vi "Thumper Control.vi"(11 "Thump":bool) -> ()   [LabVIEW 2016]
uses:
  <vilib>/Rock Robotics/Network Tables/NT Read Number.vi
  <vilib>/Rock Robotics/WPI/Solenoid/WPI_SolenoidSetEnum.vi
  <vilib>/Rock Robotics/WPI/Solenoid/Deprecated/WPI_SolenoidGetBool.vi
panel:
  in  "Thumper Status":bool
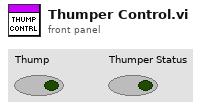
[diagram p1: front panel]
types:
  T1 = typedef "WPI_SolenoidDevRef.ctl" = cluster{"DevStatus":errorcluster, "Pneumatics Control Module":u8, "Forward Solenoid Channel":T2, "Reverse Solenoid Channel":T2}
  T2 = typedef "WPI_SolenoidChannel.ctl" = enum8{"Solenoid 0", "Solenoid 1", "Solenoid 2", "Solenoid 3", "Solenoid 4", "Solenoid 5", "Solenoid 6", "Solenoid 7", "Invalid"}
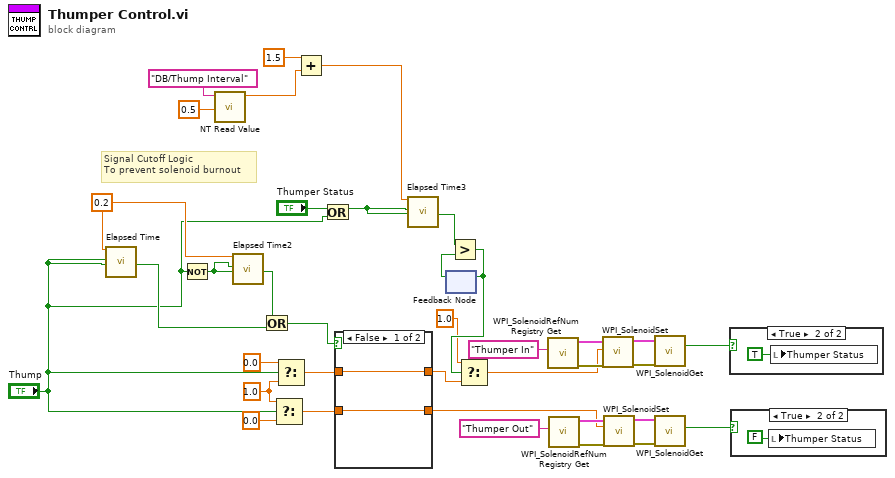
[diagram p0: block diagram]
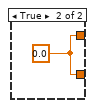
[diagram p4: hidden frame]
diagram:
  w31 = 0.2 ("Time Target (s)")
  w26 = 1.0 ("f")
  # "Signal Cutoff Logic\nTo prevent solenoid burnout"
  n1 = call "Elapsed Time"("Time Target (s)"=w31, "Reset"="Thump", "Auto Reset"="Thump") -> ("Time has Elapsed"=w28:bool)  [unwired: 9 in, 7 out]
  n2 = Not(x="Thump") -> (.not. x?=w30:bool)
  n3 = call-poly <vilib>:"NT Read Value.vi"("Default Value"=0.5, "Name"="DB/Thump Interval") -> ("Numeric"=w5:dbl)  [unwired: 8 in, 1 out]
  n4 = call "Elapsed Time2"("Time Target (s)"=w31, "Reset"=w30, "Auto Reset"=w30) -> ("Time has Elapsed"=w29:bool)  [unwired: 9 in, 7 out]
  n5 = Or(x=w29, y=w28) -> (x .or. y?=w27:bool)
  n6 = Select(t=w26, s="Thump", f=0.0) -> (s? t:f=w24:dbl)
  n7 = Select(t=0.0, s="Thump", f=w26) -> (s? t:f=w23:dbl)
  n8 = Add(x=1.5 ("Time Target (s)"), y=w5) -> (x+y=w4:dbl)
  n9 = Or(x="Thumper Status", y="Thump") -> (x .or. y?=w2:bool)
  n10 = case shown="False" w27 {
    tunnel: [w39 w40] -> w25
    tunnel: w24 -> [w39 _]
    tunnel: [w38 w40] -> w13
    tunnel: w23 -> [w38 _]
    frame False {
    }
    frame True {
      w40 = 0.0 ("f")
    }
  }
  n11 = call "Elapsed Time3"("Time Target (s)"=w4, "Reset"=w2, "Auto Reset"=w2) -> ("Time has Elapsed"=w12:bool)  [unwired: 9 in, 7 out]
  n12 = feedback #1() -> (w11:bool)  [unwired: 1 in]
  n13 = Greater?(x=w12, y=w11) -> (0:w10:bool)
  n14 = feedback-in #1(w10) -> ()
  n15 = Select(t=1.0, s=w10, f=w13) -> (s? t:f=w14:dbl)
  n16 = call <vilib>:"WPI_SolenoidRefNum Registry Get.vi"("refnum name"="Thumper In") -> ("error out"=w37:errorcluster, "SolenoidDevRef"=w36:T1)  [unwired: 9 in]
  n17 = call <vilib>:"WPI_SolenoidRefNum Registry Get.vi"("refnum name"="Thumper Out") -> ("error out"=w34:errorcluster, "SolenoidDevRef"=w33:T1)  [unwired: 9 in]
  n18 = call-poly <vilib>:"WPI_SolenoidSet.vi"("error in (no error)"=w37, "Value"=w14, "SolenoidDevRef"=w36) -> ("error out"=w20:errorcluster, "SolenoidDevRef"=w19:T1)  [unwired: 7 in]
  n19 = call-poly <vilib>:"WPI_SolenoidSet.vi"("error in (no error)"=w34, "Value"=w25, "SolenoidDevRef"=w33) -> ("error out"=w18:errorcluster, "SolenoidDevRef"=w17:T1)  [unwired: 7 in]
  n20 = call-poly <vilib>:"WPI_SolenoidGet.vi"("error in (no error)"=w20, "SolenoidDevRef"=w19) -> ("Value"=w15:bool)  [unwired: 7 in, 2 out]
  n21 = call-poly <vilib>:"WPI_SolenoidGet.vi"("error in (no error)"=w18, "SolenoidDevRef"=w17) -> ("Value"=w16:bool)  [unwired: 7 in, 2 out]
  n22 = case shown="True" w15 {
    frame False {
    }
    frame True {
      n23 = local write "Thumper Status"(TRUE) -> ()
    }
  }
  n24 = case shown="True" w16 {
    frame False {
    }
    frame True {
      n25 = local write "Thumper Status"(FALSE) -> ()
    }
  }
